vi "Queue Driver.vi"(0 "Name":string, 5 "Status":string, 7 "Status Array":string[](array[string]), 11 "Error In":errorcluster, 14 "Queue operation":T1) -> (4 "Dequeued status":string, 15 "Error Out":errorcluster)   [LabVIEW 2020]
doc: "This Queue Driver is used to create,enqueue and dequeue to the queue"
uses:
  Assignment 14/Car Wash/CarWash/Typedefs/Queue Operations.ctl
panel:
  # "This Queue Driver is used to create,enqueue and dequeue to the queue"
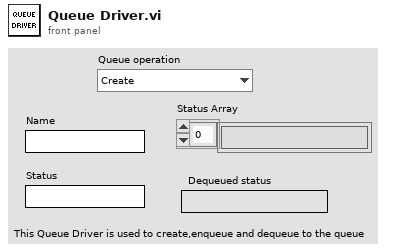
[diagram p1: front panel]
types:
  T1 = typedef "Queue Operations.ctl" = enum16{"Create", "Enqueue", "Enqueue N elements", "Enstack", "Enstack N elements", "Dequeue", "Flush queue", "Release queue"}
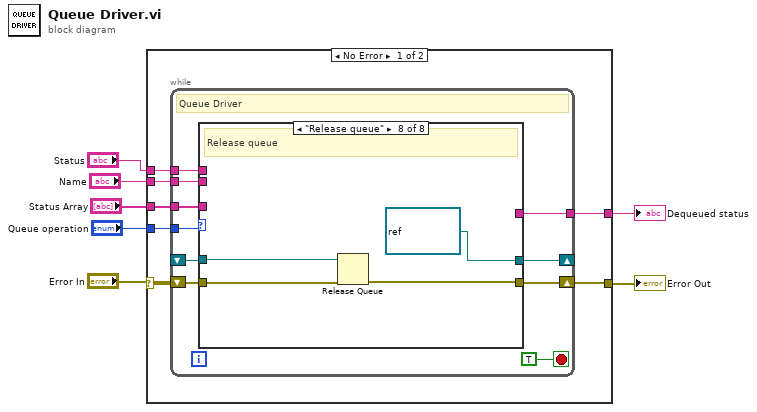
[diagram p0: block diagram]
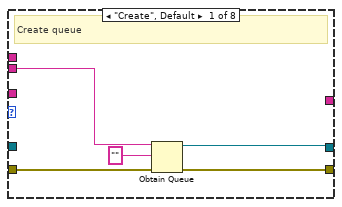
[diagram p2: hidden frame]
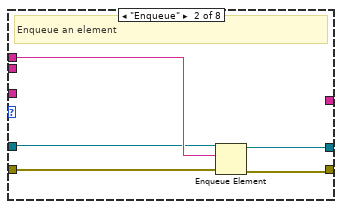
[diagram p3: hidden frame]
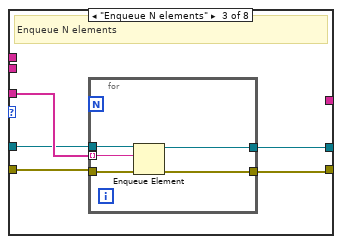
[diagram p4: hidden frame]
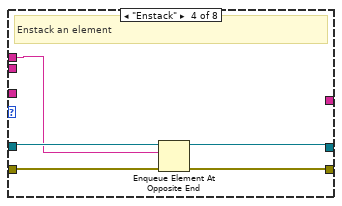
[diagram p5: hidden frame]
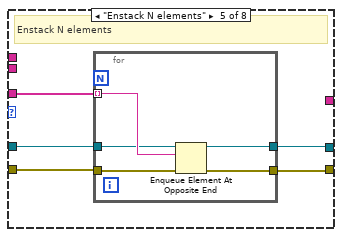
[diagram p6: hidden frame]
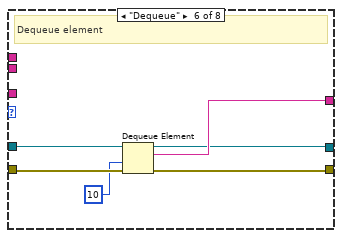
[diagram p7: hidden frame]
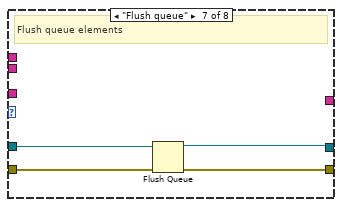
[diagram p8: hidden frame]
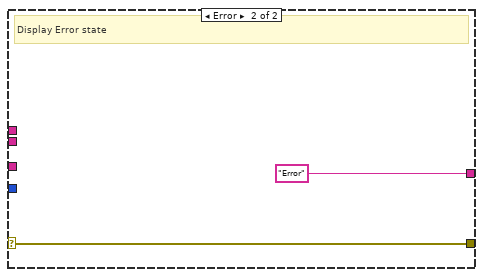
[diagram p9: hidden frame]
diagram:
  n1 = case shown="No Error" "Error In" {
    selector: "Error In" -> [w11 w75]
    tunnel: [w10 w75] -> w7
    tunnel: "Queue operation" -> [w14 _]
    tunnel: "Status Array" -> [w13 _]
    tunnel: "Name" -> [w12 _]
    tunnel: [w9 "Error"] -> w2
    tunnel: "Status" -> [w8 _]
    frame No Error {
      n2 = while {
        tunnel: w14 -> [w24]
        tunnel: w13 -> [w23]
        shift-right: [w20] -> w10
        shift-left: w11 -> [w21]
        tunnel: w12 -> [w22]
        tunnel: [w19] -> w9
        shift-right: [w18] -> _
        shift-left: _ -> [w17]
        tunnel: w8 -> [w15]
        stop <- TRUE stop-if-true
        # "Queue Driver"
        n3 = case shown="\"Release queue\"" w24 {
          tunnel: w23 -> [_ _ w37 _ w52 _ _ _]
          tunnel: w22 -> [w27 _ _ _ _ _ _ _]
          tunnel: w21 -> [w29 w30 w39 w49 w54 w65 w69 w73]
          tunnel: [w28 w34 w38 w48 w53 w64 w68 w72] -> w20
          tunnel: [_ _ _ _ _ w63 _ _] -> w19
          tunnel: w17 -> [_ w31 w36 w46 w51 w61 w67 w70]
          tunnel: [w25 w33 w35 w47 w50 w60 w66 refnum<queue> refnum ("queue out")] -> w18
          tunnel: w15 -> [_ w32 _ w45 _ _ _ _]
          frame "Create", Default {
            # "Create queue"
            n4 = Obtain Queue(name (unnamed)=w27, element data type="", error in (no error)=w29) -> (queue out=w25:refnum<queue>, error out=w28:errorcluster)  [unwired: 2 in, 1 out]
          }
          frame "Enqueue" {
            # "Enqueue an element"
            n5 = Enqueue Element(queue=w31, element=w32, error in (no error)=w30) -> (queue out=w33:refnum<queue>, error out=w34:errorcluster)  [unwired: 1 in, 1 out]
          }
          frame "Enqueue N elements" {
            # "Enqueue N elements"
            n6 = for {
              tunnel: w37 -> [w42] mode=indexing
              tunnel: w39 -> [w44]
              tunnel: [w43] -> w38
              tunnel: [w41] -> w35
              tunnel: w36 -> [w40]
              n7 = Enqueue Element(queue=w40, element=w42, error in (no error)=w44) -> (queue out=w41:refnum<queue>, error out=w43:errorcluster)  [unwired: 1 in, 1 out]
            }
          }
          frame "Enstack" {
            # "Enstack an element"
            n8 = Enqueue Element At Opposite End(queue=w46, element=w45, error in (no error)=w49) -> (queue out=w47:refnum<queue>, error out=w48:errorcluster)  [unwired: 1 in, 1 out]
          }
          frame "Enstack N elements" {
            # "Enstack N elements"
            n9 = for {
              tunnel: [w57] -> w50
              tunnel: w54 -> [w59]
              tunnel: [w58] -> w53
              tunnel: w52 -> [w56] mode=indexing
              tunnel: w51 -> [w55]
              n10 = Enqueue Element At Opposite End(queue=w55, element=w56, error in (no error)=w59) -> (queue out=w57:refnum<queue>, error out=w58:errorcluster)  [unwired: 1 in, 1 out]
            }
          }
          frame "Dequeue" {
            # "Dequeue element"
            n11 = Dequeue Element(queue=w61, timeout in ms (-1)=10, error in (no error)=w65) -> (queue out=w60:refnum<queue>, element=w63:string, error out=w64:errorcluster)  [unwired: 1 out]
          }
          frame "Flush queue" {
            # "Flush queue elements"
            n12 = Flush Queue(queue=w67, error in (no error)=w69) -> (queue out=w66:refnum<queue>, error out=w68:errorcluster)  [unwired: 1 out]
          }
          frame "Release queue" {
            # "Release queue"
            n13 = Release Queue(queue=w70, error in (no error)=w73) -> (error out=w72:errorcluster)  [unwired: 1 in, 2 out]
          }
        }
      }
    }
    frame Error {
      # "Display Error state"
    }
  }
  "Error Out" <- w7
  "Dequeued status" <- w2
